vi "Letter Statistics.vi"(11 "Dictionary":string[](array[string])) -> (3 "Statistic":T1[](array[typedef]))   [LabVIEW 2015]
uses:
  TypeDef/Letter Statistic.ctl
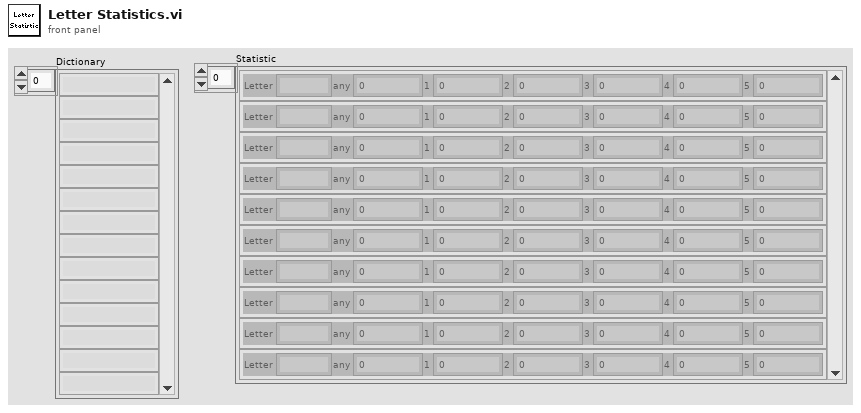
[diagram p1: front panel]
types:
  T1 = typedef "Letter Statistic.ctl" = cluster{"Letter":string, "any":dbl, "1":dbl, "2":dbl, "3":dbl, "4":dbl, "5":dbl}
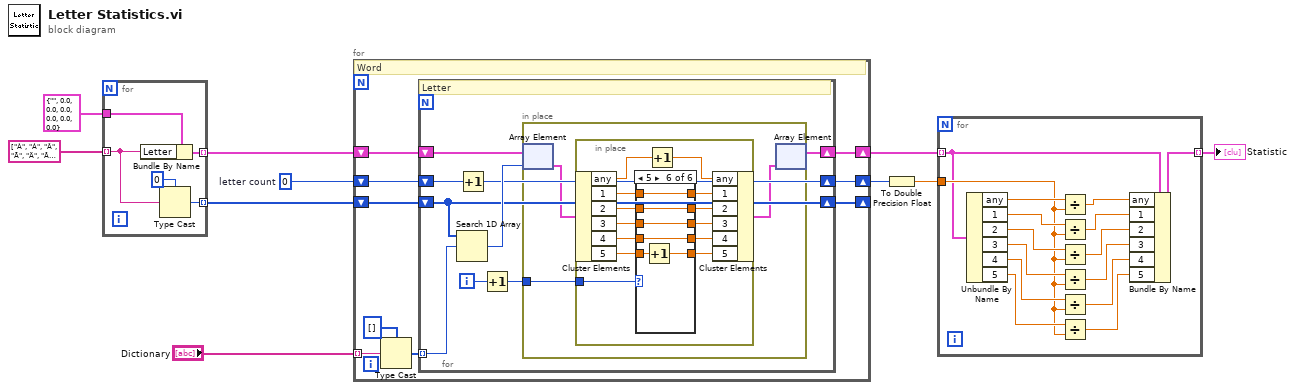
[diagram p0: block diagram]
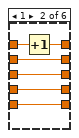
[diagram p3: hidden frame]
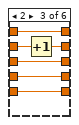
[diagram p4: hidden frame]
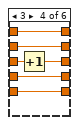
[diagram p5: hidden frame]
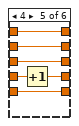
[diagram p6: hidden frame]
diagram:
  w9 = u64 0  # letter count
  n1 = for {
    tunnel: string[] ["À", "Á", "Â", "Ã", "Ä", "Å", "Æ", "Ç", "È", "É", "Ê", "Ë", "Ì", "Í", "Î", "Ï", "Ð", "Ñ", "Ò", "Ó", "Ô", "Õ", "Ö", "×", "Ø", "Ù", "Ú", "Û", "Ü", "Ý", "Þ", "ß"] ("Letter") -> [w13] mode=indexing
    tunnel: T1 {"Letter"="", "any"=0.0, "1"=0.0, "2"=0.0, "3"=0.0, "4"=0.0, "5"=0.0} ("Letter Statistic") -> [w15]
    tunnel: [w14] -> w2 mode=indexing
    tunnel: [w11] -> w1 mode=indexing
    n2 = Bundle By Name(cluster=w15, "Letter"=w13) -> (w14:T1)
    n3 = Type Cast(type=u8 0, x=w13) -> (*(type *) &x=w11:u8)
  }
  n4 = for {
    tunnel: "Dictionary" -> [w20] mode=indexing
    shift-right: [w23] -> w5
    shift-left: w2 -> [w24]
    shift-right: [w21] -> w8
    shift-left: w9 -> [w22]
    shift-right: [w18] -> _
    shift-left: w1 -> [w19]
    # "Word"
    n5 = Type Cast(type=u8[] [] ("letter"), x=w20) -> (*(type *) &x=w17:u8[])
    n6 = for {
      shift-right: [w31] -> w23
      shift-left: w24 -> [w27]
      shift-right: [w29] -> w21
      shift-left: w22 -> [w26]
      tunnel: w17 -> [w33] mode=indexing
      shift-right: [w25] -> w18
      shift-left: w19 -> [w25]
      i -> [w30]
      # "Letter"
      n7 = Search 1D Array(1D array=w25, element=w33) -> (index of element=w32:i32)  [unwired: 1 in]
      n8 = Increment(x=w26) -> (x+1=w29:u64)
      n9 = Increment(x=w30) -> (x+1=w28:i32)
      n10 = in-place {
        in-place-border: w28 -> [w34]
        n11 = in-place-array #1(w27, w32) -> (w36:T1)
        n12 = in-place {
          in-place-border: w34 -> [w47]
          n13 = in-place-cluster #2(w36) -> ("any"=w49:dbl, "1"=w46:dbl, "2"=w44:dbl, "3"=w42:dbl, "4"=w40:dbl, "5"=w38:dbl)
          n14 = case shown="5" w47 {
            tunnel: w46 -> [w50 w60 w66 w72 w78 w84]
            tunnel: [w50 w55 w66 w72 w78 w84] -> w45
            tunnel: w44 -> [w54 w56 w63 w70 w75 w82]
            tunnel: [w54 w56 w61 w70 w75 w82] -> w43
            tunnel: w42 -> [w53 w59 w62 w69 w74 w81]
            tunnel: [w53 w59 w62 w67 w74 w81] -> w41
            tunnel: w40 -> [w52 w58 w65 w68 w77 w80]
            tunnel: [w52 w58 w65 w68 w73 w80] -> w39
            tunnel: w38 -> [w51 w57 w64 w71 w76 w83]
            tunnel: [w51 w57 w64 w71 w76 w79] -> w37
            frame 0, Default {
            }
            frame 1 {
              n15 = Increment(x=w60) -> (x+1=w55:dbl)
            }
            frame 2 {
              n16 = Increment(x=w63) -> (x+1=w61:dbl)
            }
            frame 3 {
              n17 = Increment(x=w69) -> (x+1=w67:dbl)
            }
            frame 4 {
              n18 = Increment(x=w77) -> (x+1=w73:dbl)
            }
            frame 5 {
              n19 = Increment(x=w83) -> (x+1=w79:dbl)
            }
          }
          n20 = Increment(x=w49) -> (x+1=w48:dbl)
          n21 = in-place-cluster #2("any"=w48, "1"=w45, "2"=w43, "3"=w41, "4"=w39, "5"=w37) -> (w35:T1)
        }
        n22 = in-place-array #1(w35) -> (w31:T1[])  [unwired: 1 out]
      }
    }
  }
  n23 = To Double Precision Float(number=w8) -> (double precision float=w7:dbl)
  n24 = for {
    tunnel: w5 -> [w86] mode=indexing
    tunnel: w7 -> [w92]
    tunnel: [w85] -> w6 mode=indexing
    n25 = Unbundle By Name(w86) -> ("any"=w99:dbl, "1"=w97:dbl, "2"=w96:dbl, "3"=w95:dbl, "4"=w94:dbl, "5"=w93:dbl)
    n26 = Divide(x=w99, y=w92) -> (x/y=w98:dbl)
    n27 = Divide(x=w97, y=w92) -> (x/y=w91:dbl)
    n28 = Divide(x=w96, y=w92) -> (x/y=w90:dbl)
    n29 = Divide(x=w95, y=w92) -> (x/y=w89:dbl)
    n30 = Divide(x=w94, y=w92) -> (x/y=w88:dbl)
    n31 = Divide(x=w93, y=w92) -> (x/y=w87:dbl)
    n32 = Bundle By Name(cluster=w86, "any"=w98, "1"=w91, "2"=w90, "3"=w89, "4"=w88, "5"=w87) -> (w85:T1)
  }
  "Statistic" <- w6
